vi "Destroy User Events.vi"(11 "Accelerometer in":refnum<class "Accelerometer.lvclass">) -> (3 "Accelerometer out":refnum<class "Accelerometer.lvclass">)   [LabVIEW 2020, in "Accelerometer.lvlib" / "Accelerometer.lvclass"]
uses:
  Accelerometer.lvclass
  Accelerometer.lvclass/Accelerometer.ctl
  <instrlib>/Phidgets/Phidget Accelerometer/Public/AccelerometerClose.vi
  <instrlib>/Phidgets/Phidget Accelerometer/Phidget Accelerometer.lvlib
  <instrlib>/Phidgets/Phidget Common/Phidget Common.lvlib
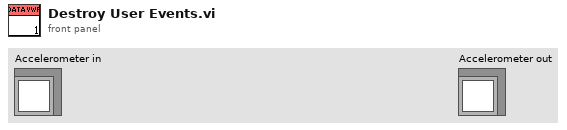
[diagram p1: front panel]
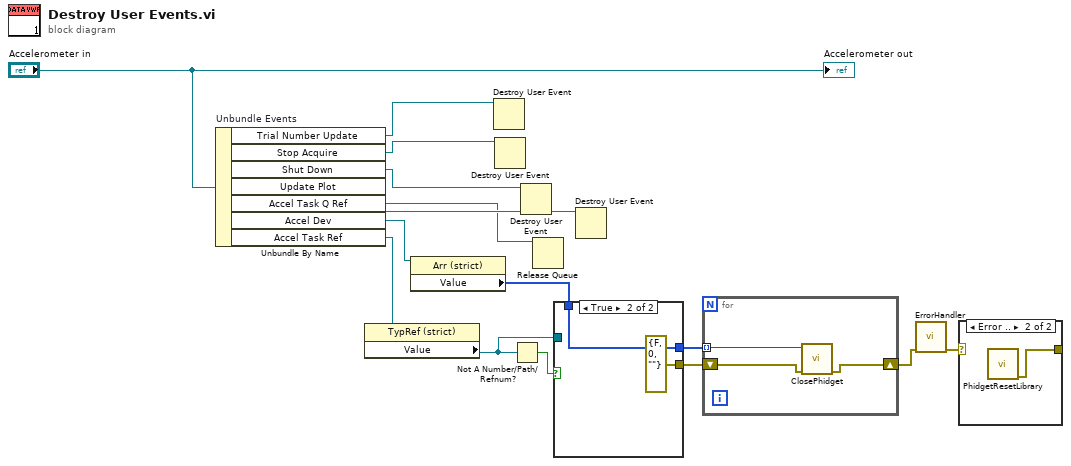
[diagram p0: block diagram]
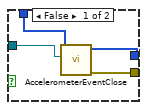
[diagram p2: hidden frame]
diagram:
  n1 = Unbundle By Name "Unbundle Events"("Accelerometer in") -> ("Trial Number Update"=w14:refnum<user-event>, "Stop Acquire"=w13:refnum<user-event>, "Shut Down"=w12:refnum<user-event>, "Update Plot"=w11:refnum<user-event>, "Accel Task Q Ref"=w10:refnum<queue>, "Accel Dev"=w9:refnum<vi>, "Accel Task Ref"=w3:refnum<vi>)
  n2 = property class="TypRef (strict)"(reference=w3) -> ("Value"=w1:refnum<event-registration>)  [unwired: 1 in, 2 out]
  n3 = property class="Arr (strict)"(reference=w9) -> ("Value"=w6:u64[])  [unwired: 1 in, 2 out]
  n4 = Destroy User Event(user event=w14) -> ()  [unwired: 1 in, 1 out]
  n5 = Destroy User Event(user event=w13) -> ()  [unwired: 1 in, 1 out]
  n6 = Not A Number/Path/Refnum?(number/path/refnum=w1) -> (NaN/Path/Refnum?=w2:bool)
  n7 = Destroy User Event(user event=w12) -> ()  [unwired: 1 in, 1 out]
  n8 = Release Queue(queue=w10) -> ()  [unwired: 2 in, 3 out]
  n9 = case shown="True" w2 {
    tunnel: [w19 w21] -> w8
    tunnel: [w18 errorcluster {"status"=FALSE, "code"=0, "source"=""} ("error out")] -> w7
    tunnel: w6 -> [w17 w21]
    tunnel: w1 -> [w16 _]
    frame False {
      n10 = call <instrlib>:"AccelerometerEventClose.vi"("Event Registration Refnum In"=w16, "Devices In"=w17) -> ("error out"=w18:errorcluster, "Devices Out"=w19:u64[])  [unwired: 8 in]
    }
    frame True {
    }
  }
  n11 = Destroy User Event(user event=w11) -> ()  [unwired: 1 in, 1 out]
  n12 = for {
    tunnel: w8 -> [w24] mode=indexing
    shift-right: [w22] -> w4
    shift-left: w7 -> [w23]
    n13 = call-poly <instrlib>:"ClosePhidget.vi"("error in"=w23, "Device In"=w24) -> ("error out"=w22:errorcluster)  [unwired: 9 in]
  }
  n14 = call <instrlib>:"ErrorHandler.vi"("error in"=w4) -> ("error out"=w5:errorcluster)  [unwired: 9 in, 1 out]
  n15 = case shown="Error .." w5 {
    selector: w5 -> [w25 _]
    tunnel: [w25 w26] -> _
    frame No Error {
    }
    frame Error {
      n16 = call <instrlib>:"PhidgetResetLibrary.vi"() -> ("error out"=w26:errorcluster)  [unwired: 11 in]
    }
  }
  "Accelerometer out" <- "Accelerometer in"
